vi "Auto Drive.vi"() -> ()   [LabVIEW 2018]
uses:
  Robot Global Data.vi
  AppleScript/Apple script.lvlib
panel:
  in  "Cluster 5":T1={"kp"=0.45, "ki"=0.0005, "kd"=0.017, "kv"=0.102, "ka"=0.035}
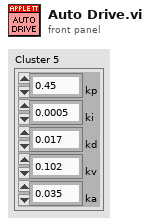
[diagram p1: front panel]
types:
  T1 = cluster{"kp":dbl, "ki":dbl, "kd":dbl, "kv":dbl, "ka":dbl}
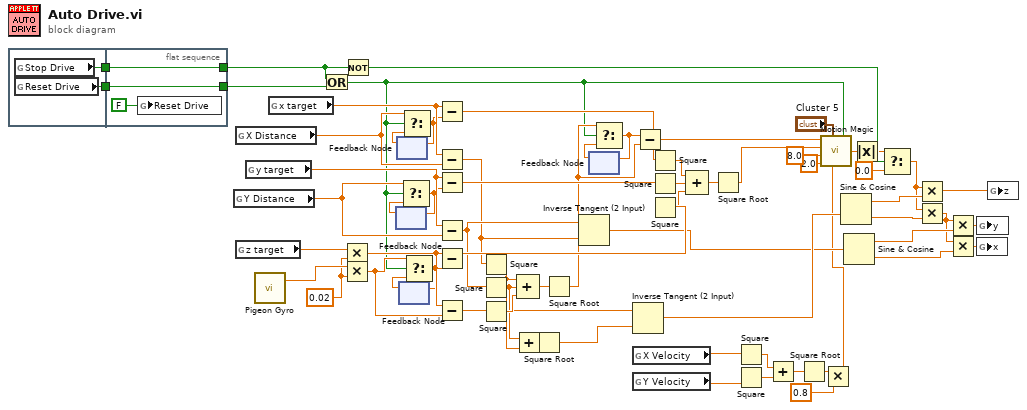
[diagram p0: block diagram]
diagram:
  w46 = 0.02 ("y")
  n1 = flat-sequence {
    tunnel: [w69] -> w67
    tunnel: [w68] -> w66
    tunnel: [w72] -> w64
    tunnel: [w70] -> w65
    tunnel: w67 -> [w70]
    tunnel: w66 -> [w72]
    frame #0 {
      n2 = global read "Robot Global Data.vi" "Stop Drive"() -> (w68:bool)
      n3 = global read "Robot Global Data.vi" "Reset Drive"() -> (w69:bool)
    }
    frame #1 {
      n4 = global write "Robot Global Data.vi" "Reset Drive"(FALSE ("top rive")) -> ()
    }
  }
  n5 = global read "Robot Global Data.vi" "Y Distance"() -> (w7:dbl)
  n6 = global read "Robot Global Data.vi" "X Distance"() -> (w11:dbl)
  n7 = global read "Robot Global Data.vi" "z target"() -> (w53:dbl)
  n8 = global read "Robot Global Data.vi" "y target"() -> (w43:dbl)
  n9 = call "Pigeon Gyro.vi"() -> ("YPR.Yaw"=w47:dbl)  [unwired: 2 in, 1 out]
  n10 = global read "Robot Global Data.vi" "x target"() -> (w44:dbl)
  n11 = Or(x=w64, y=w65) -> (x .or. y?=w5:bool)
  n12 = Multiply(x=w53, y=w46) -> (x*y=w42:dbl)
  n13 = Multiply(x=w47, y=w46) -> (x*y=w6:dbl)
  n14 = Not(x=w64) -> (.not. x?=w56:bool)
  n15 = feedback #1() -> (w8:dbl)  [unwired: 1 in]
  n16 = feedback #2() -> (w12:dbl)  [unwired: 1 in]
  n17 = feedback #3() -> (w4:dbl)  [unwired: 1 in]
  n18 = Select(t=w7, s=w5, f=w8) -> (s? t:f=w9:dbl)
  n19 = feedback-in #1(w9) -> ()
  n20 = Select(t=w11, s=w5, f=w12) -> (s? t:f=w10:dbl)
  n21 = feedback-in #2(w10) -> ()
  n22 = Select(t=w6, s=w5, f=w4) -> (s? t:f=w3:dbl)
  n23 = feedback-in #3(w3) -> ()
  n24 = Subtract(x=w44, y=w10) -> (x-y=w31:dbl)
  n25 = Subtract(x=w44, y=w11) -> (x-y=w16:dbl)
  n26 = Subtract(x=w43, y=w9) -> (x-y=w27:dbl)
  n27 = Subtract(x=w43, y=w7) -> (x-y=w18:dbl)
  n28 = Subtract(x=w42, y=w3) -> (x-y=w29:dbl)
  n29 = Subtract(x=w42, y=w6) -> (x-y=w19:dbl)
  n30 = Square(x=w16) -> (x^2=w24:dbl)
  n31 = Square(x=w18) -> (x^2=w23:dbl)
  n32 = Square(x=w19) -> (x^2=w26:dbl)
  n33 = Add(x=w23, y=w24) -> (x+y=w21:dbl)
  n34 = Compound Arithmetic op=ADD(w24, w23, w26) -> (w25:dbl)
  n35 = Square Root(x=w21) -> (sqrt(x)=w20:dbl)
  n36 = Square Root(x=w25) -> (sqrt(x)=w15:dbl)
  n37 = Inverse Tangent (2 Input)(1:w16, 2:w18) -> (0:w17:dbl)
  n38 = feedback #4() -> (w13:dbl)  [unwired: 1 in]
  n39 = Select(t=w15, s=w5, f=w13) -> (s? t:f=w14:dbl)
  n40 = feedback-in #4(w14) -> ()
  n41 = Inverse Tangent (2 Input)(1:w20, 2:w19) -> (0:w22:dbl)
  n42 = global read "Robot Global Data.vi" "X Velocity"() -> (w37:dbl)
  n43 = global read "Robot Global Data.vi" "Y Velocity"() -> (w36:dbl)
  n44 = Subtract(x=w14, y=w15) -> (x-y=w41:dbl)
  n45 = Square(x=w31) -> (x^2=w33:dbl)
  n46 = Square(x=w27) -> (x^2=w32:dbl)
  n47 = Square(x=w29) -> (x^2=w28:dbl)
  n48 = Compound Arithmetic op=ADD(w33, w32, w28) -> (w34:dbl)
  n49 = Square Root(x=w34) -> (sqrt(x)=w30:dbl)
  n50 = Square(x=w37) -> (x^2=w39:dbl)
  n51 = Square(x=w36) -> (x^2=w40:dbl)
  n52 = Add(x=w39, y=w40) -> (x+y=w38:dbl)
  n53 = Square Root(x=w38) -> (sqrt(x)=w35:dbl)
  n54 = Multiply(x=w35, y=0.8) -> (x*y=w2:dbl)
  n55 = call "Motion Magic.vi"("In"=w41, "Cluster"="Cluster 5", "Target"=w30, "Max V"=8.0, "Velocity"=w2, "Max A"=2.0, "Reset"=w5) -> ("Output"=w63:dbl)  [unwired: 1 out]
  n56 = Sine & Cosine(0:w22) -> (1:w49:dbl, 2:w50:dbl)
  n57 = Sine & Cosine(0:w17) -> (1:w60:dbl, 2:w58:dbl)
  n58 = Absolute Value(x=w63) -> (abs(x)=w45:dbl)
  n59 = Select(t=w45, s=w56, f=0.0) -> (s? t:f=w48:dbl)
  n60 = Multiply(x=w48, y=w49) -> (x*y=w52:dbl)
  n61 = Multiply(x=w48, y=w50) -> (x*y=w51:dbl)
  n62 = Multiply(x=w51, y=w60) -> (x*y=w59:dbl)
  n63 = Multiply(x=w51, y=w58) -> (x*y=w57:dbl)
  n64 = global write "Robot Global Data.vi" "y"(w59) -> ()
  n65 = global write "Robot Global Data.vi" "x"(w57) -> ()
  n66 = global write "Robot Global Data.vi" "z"(w52) -> ()
